vi "Save Image.vi"(8 "error in (no error)":errorcluster, 9 "Save Path":path, 10 "Image":T1, 11 "Imaq Camera in":refnum<class "Imaq Camera.lvclass">) -> (0 "error out":errorcluster, 3 "Imaq Camera out":refnum<class "Imaq Camera.lvclass">)   [LabVIEW 2022 SP3, in "Imaq Camera.lvclass"]
uses:
  Imaq Camera.lvclass
  <vilib>/vision/Image Controls.llb/IMAQ Image.ctl
  Imaq Camera.lvclass/Imaq Camera.ctl
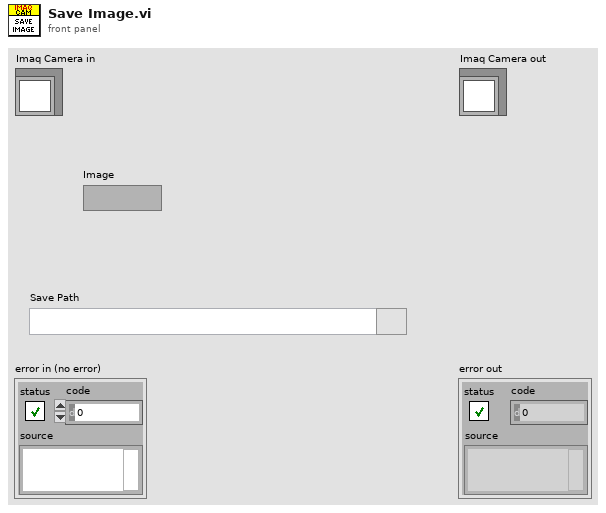
[diagram p1: front panel]
types:
  T1 = typedef "IMAQ Image.ctl" = refnum<image>
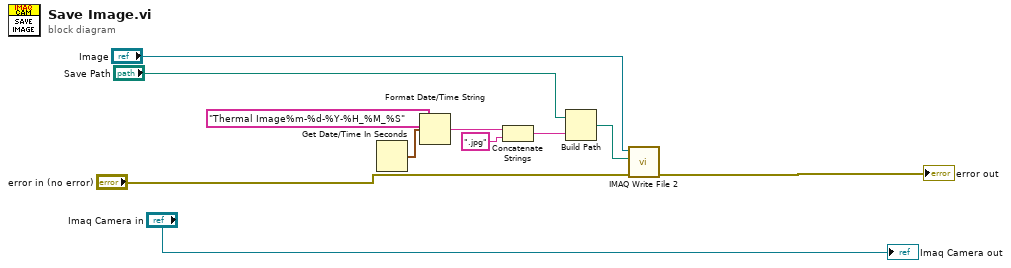
[diagram p0: block diagram]
diagram:
  n1 = Get Date/Time In Seconds() -> (seconds since 1Jan1904=w8:timestamp)
  n2 = Format Date/Time String(time format string (%c)="Thermal Image%m-%d-%Y-%H_%M_%S", seconds (now)=w8) -> (date/time string=w7:string)  [unwired: 1 in]
  n3 = Concatenate Strings(w7, ".jpg" ("string")) -> (w5:string)
  n4 = Build Path(base path="Save Path", name or relative path=w5) -> (appended path=w4:path)
  n5 = call-poly "IMAQ Write File 2"("error in (no error)"="error in (no error)", "File Path"=w4, "Image"="Image") -> ("error out"=→"error out":errorcluster)  [unwired: 7 in, 1 out]
  "Imaq Camera out" <- "Imaq Camera in"
